vi "vision1.vi"(0 "Color Plane (Color Plane Extraction 1)":i32(ring)=2 items=["Red", "Green", "Blue", "Hue", "Saturation", "Luminance", "Value", "Intensity"], 1 "Range (Threshold 1)":cluster{"Lower value":sgl, "Upper value":sgl}={"Lower value"=199.0, "Upper value"=255.0}, 2 "Number of Erosion (Adv. Morphology 1)":i32=1, 3 "Square/Hexa (Square) (Adv. Morphology 1)":bool, 4 "Connectivity 4/8 (8) (Adv. Morphology 1)":bool=TRUE, 5 "Low Pass/High Pass (Low) (Adv. Morphology 1)":bool, 7 "error in":errorcluster) -> (20 "Number of Matches (Shape Matching 1)":i32, 21 "Shape Report (calibrated) (Shape Matching 1)":T2(array[cluster]) {"Score" format="%.2f"; "Centroid"."y" format="%.2f"; "Centroid"."x" format="%.2f"}, 22 "Centroid (Centroid 1)":cluster{"X Centroid":sgl, "Y Centroid":sgl} {"Y Centroid" format="%.2f"; "X Centroid" format="%.2f"}, 23 "Calibrated Centroid (Centroid 1)":cluster{"X Centroid":sgl, "Y Centroid":sgl} {"Y Centroid" format="%.2f"; "X Centroid" format="%.2f"}, 27 "error out":errorcluster)   [LabVIEW 2016]
uses:
  <vilib>/vision/driver/NI_Vision_Acquisition_Software.lvlib
  <vilib>/vision/NI_Vision_Development_Module.lvlib
panel:
  out "Image Out":T1(plugin-control)
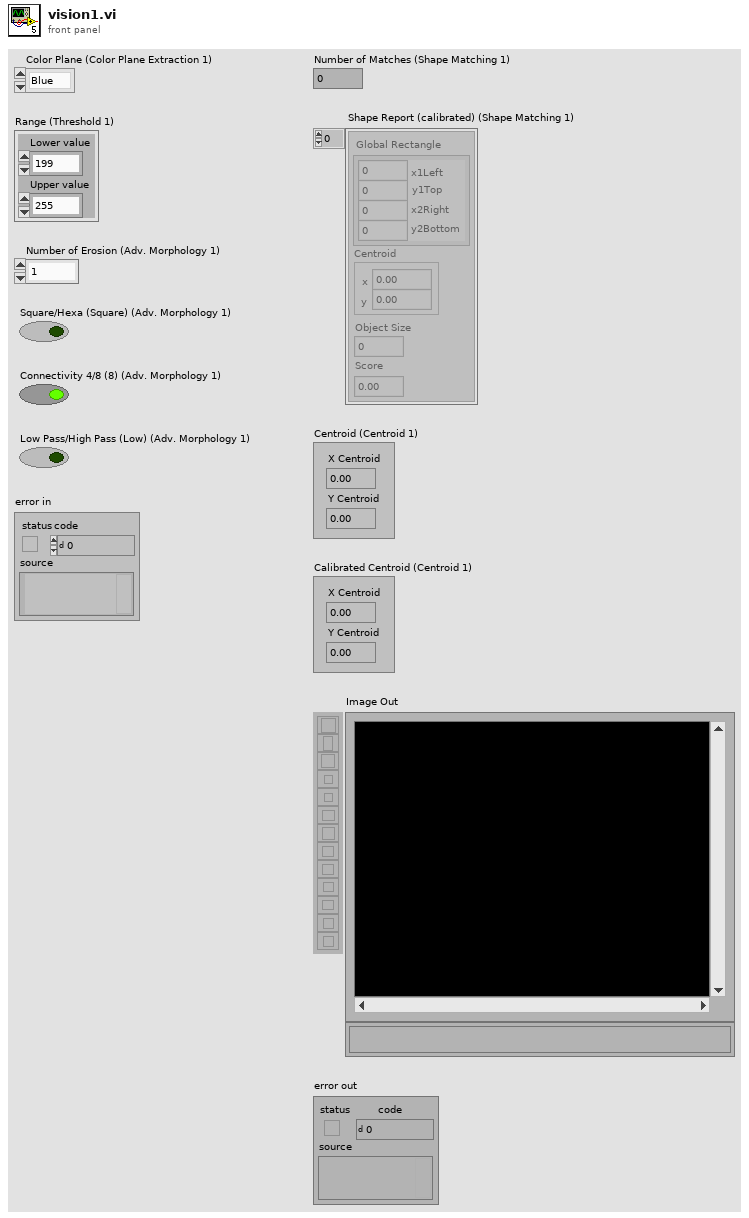
[diagram p1: front panel]
types:
  T1 = typedef "IMAQ Image.ctl" = refnum<image>
  T2 = cluster{"Global Rectangle":cluster{"x1Left":i32, "y1Top":i32, "x2Right":i32, "y2Bottom":i32}, "Centroid":cluster{"x":sgl, "y":sgl}, "Object Size":u32, "Score":dbl}[]
  T3 = typedef "IMAQdx.ctl" = refnum<k21>
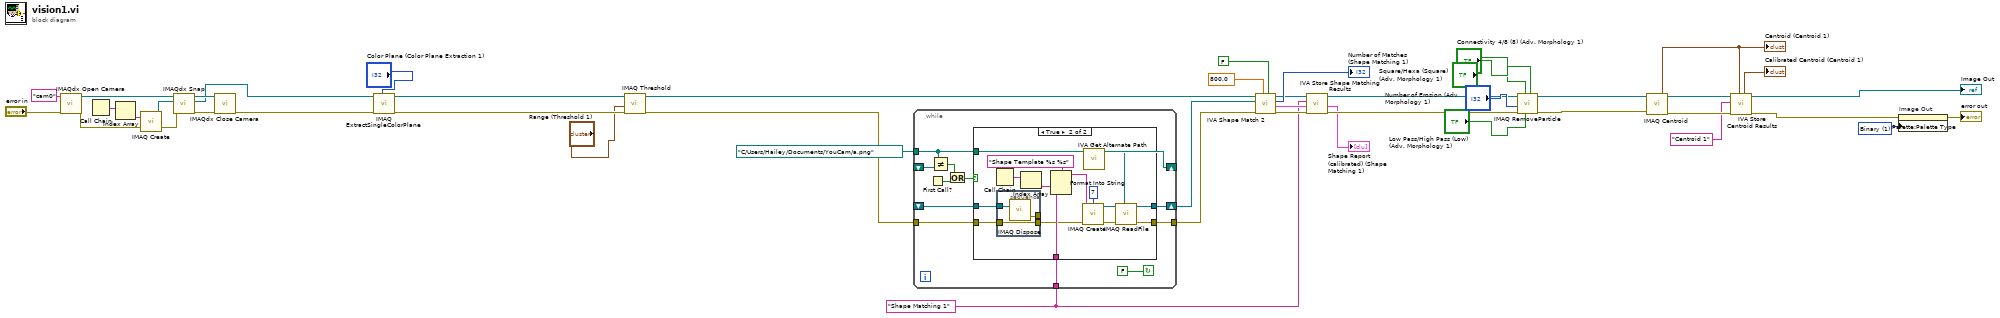
[diagram p0: block diagram]
diagram:
  w1 = u32 1 items=["Grayscale", "Binary", "Gradient", "Rainbow", "Temperature", "User Defined", "Binary 16 Bit", "Gradient 16 Bit", "Rainbow 16 Bit", "Temperature 16 Bit", "User Defined 16 Bit"] ("Palette Type")
  w16 = "Shape Matching 1" ("Step Name")
  n1 = call <vilib>:"IMAQdx Open Camera.vi"("error in"="error in", "Session In"="cam0" ("Interface Name")) -> ("error out"=w44:errorcluster, "Session Out"=w38:T3)  [unwired: 1 in, 7 out]
  n2 = Call Chain() -> (call chain=w36:string[])
  n3 = Index Array(array=w36) -> (element=w35:string)  [unwired: 1 in]
  n4 = call "IMAQ Create"("Image Name"=w35, "error in (no error)"=w44) -> ("New Image"=w40:T1, "error out"=w39:errorcluster)  [unwired: 2 in, 1 out]
  n5 = call <vilib>:"IMAQdx Snap.vi"("error in"=w39, "Image In"=w40, "Session In"=w38) -> ("error out"=w42:errorcluster, "Image Out"=w33:T1, "Session Out"=w43:T3)  [unwired: 6 out]
  n6 = call <vilib>:"IMAQdx Close Camera.vi"("error in"=w42, "Session In"=w43) -> ("error out"=w41:errorcluster)  [unwired: 9 out]
  n7 = call "IMAQ ExtractSingleColorPlane"("Color Plane"="Color Plane (Color Plane Extraction 1)", "error in (no error)"=w41, "Image Src"=w33) -> ("error out"=w32:errorcluster, "Image Dst Out"=w30:T1)  [unwired: 1 in, 6 out]
  n8 = call "IMAQ Threshold"("error in (no error)"=w32, "Range"="Range (Threshold 1)", "Image Src"=w30) -> ("error out"=w29:errorcluster, "Image Dst Out"=w25:T1)  [unwired: 3 in, 4 out]
  n9 = while {
    shift-right: [w56] -> w17
    shift-left: _ -> [w55]
    tunnel: [w53] -> w18
    tunnel: w29 -> [w52]
    tunnel: path "C:/Users/Hailey/Documents/YouCam/a.png" ("Template Path") -> [w50]
    tunnel: w16 -> [w51]
    shift-right: [w50] -> _
    shift-left: _ -> [w49]
    stop <- FALSE continue-if-true
    n10 = First Call?() -> (First Call?: T/F=w48:bool)
    n11 = Not Equal?(x=w50, y=w49) -> (x != y?=w47:bool)
    n12 = Or(x=w47, y=w48) -> (x .or. y?=w46:bool)
    n13 = case shown="True" w46 {
      tunnel: [w58 w70] -> w56
      tunnel: w55 -> [w58 w61]
      tunnel: [w57 w68] -> w53
      tunnel: w52 -> [w57 w60]
      tunnel: w50 -> [_ w63]
      tunnel: w51 -> [_ w64]
      frame False {
      }
      frame True {
        n14 = Call Chain() -> (call chain=w66:string[])
        n15 = stacked-sequence {
          tunnel: w61 -> [w76]
          tunnel: w60 -> [w75]
          tunnel: [w75] -> w59
          tunnel: [w74] -> _
          frame #0 {
            n16 = call "IMAQ Dispose"("Image"=w76) -> ("error out"=w74:errorcluster)  [unwired: 2 in, 3 out]
          }
        }
        n17 = Index Array(array=w66) -> (element=w65:string)  [unwired: 1 in]
        n18 = Format Into String(format string="Shape Template %s %s" ("Image Name"), w65, w64) -> (resulting string=w73:string)  [unwired: 2 in, 1 out]
        n19 = call "IMAQ Create"("Border Size"=7, "Image Name"=w73, "error in (no error)"=w59) -> ("New Image"=w71:T1, "error out"=w69:errorcluster)  [unwired: 1 in, 1 out]
        n20 = call <vilib>:"IVA Get Alternate Path.vi"("Path In"=w63) -> ("Path Out"=w62:path)  [unwired: 10 out]
        n21 = call "IMAQ ReadFile"("File Path"=w62, "error in (no error)"=w69, "Image"=w71) -> ("error out"=w68:errorcluster, "Image Out"=w70:T1)  [unwired: 2 in, 5 out]
      }
    }
  }
  n22 = call <vilib>:"IVA Shape Match 2.vi"("Scale Invariance"=FALSE, "Minimal Score"=800.0, "error in (no error)"=w18, "Template"=w17, "Image Src"=w25) -> ("error out"=w24:errorcluster, "Shape Report"=w22:T2, "Number of Matches"=→"Number of Matches (Shape Matching 1)":i32, "Image Out"=w21:T1)  [unwired: 3 out]
  n23 = call <vilib>:"IVA Store Shape Matching Results.vi"("error in (no error)"=w24, "Shape Report"=w22, "Step Name"=w16, "Image in"=w21) -> ("error out"=w23:errorcluster, "Shape Report (calibrated)"=→"Shape Report (calibrated) (Shape Matching 1)":T2, "Image dup"=w11:T1)  [unwired: 5 out]
  n24 = call "IMAQ RemoveParticle"("Connectivity 4/8 (8)"="Connectivity 4/8 (8) (Adv. Morphology 1)", "Low Pass/High Pass (Low)"="Low Pass/High Pass (Low) (Adv. Morphology 1)", "Square/Hexa (Square)"="Square/Hexa (Square) (Adv. Morphology 1)", "error in (no error)"=w23, "Number of Erosion"="Number of Erosion (Adv. Morphology 1)", "Image Src"=w11) -> ("error out"=w10:errorcluster, "Image Dst Out"=w7:T1)  [unwired: 1 in, 3 out]
  n25 = call "IMAQ Centroid"("error in (no error)"=w10, "Image"=w7) -> ("error out"=w9:errorcluster, "Centroid"=w5:cluster{"X Centroid":sgl, "Y Centroid":sgl})  [unwired: 1 in, 1 out]
  "Centroid (Centroid 1)" <- w5
  n26 = call <vilib>:"IVA Store Centroid Results.vi"("Centroid in"=w5, "error in (no error)"=w9, "Step Name"="Centroid 1", "Image in"=w7) -> ("error out"=w8:errorcluster, "Image dup"=→"Image Out":T1, "Calibrated Centroid"=→"Calibrated Centroid (Centroid 1)":cluster{"X":sgl, "Y":sgl})  [unwired: 5 out]
  n27 = property on="Image Out" class="ImageControl"(error in=w8, "Palette:Palette Type"=w1) -> (error out=→"error out":errorcluster)  [unwired: 1 in, 1 out]
